vi "Find Unexpected Deps.vi"() -> ()   [LabVIEW 2019, in "DepsWatchToolsMenu.lvlib"]
doc: "GUI to compare LabVIEW code between currently checked out branch with any other branch or any of its commits.\n\n(c) 2024 Soliton Technologies. All rights reserved."
uses:
  DepsWatchToolsMenu.lvlib
  <vilib>/Hampel Software Engineering/Git API/Git API/GIT-api.lvclass
  <vilib>/Hampel Software Engineering/Git API/Git API/Controls/GIT-Repository States.ctl
  vi.lib/DepsWatch/DepsWatch.lvlib
  <userlib>/_OpenG.lib/file/file.llb/Valid Path - Traditional__ogtk.vi
  <userlib>/_OpenG.lib/file/file.llb/File Exists - Scalar__ogtk.vi
  vi.lib/DepsWatch/Typedefs/DepsCheckResult.ctl
panel:
  in  "Tab Control":T1(tab)=enum."Main UI"
  in  "Check Changed Libraries Only?":bool
  in  "Branch 2":string(combo)="origin/main" caption="Branch2 to Compare"
  in  "Refresh Current Branch":bool
  in  "Stop":bool
  in  "Repository Path":path
  in  "Branch1":string(combo)="origin/main" caption="Branch1 to Compare"
  in  "Compare":bool
  out "Current Branch Status":string
  out "Unexpected Deps":T2[](array[typedef])
  # "1. Checkout the branch of interest in your system using any method - Git command line, Desktop Git GUI Clients etc.,\n\n2. Specify the local Repository Path.\n\n3. Verify the current branch, its status and select a branch or commit based on the Compare Mode and click on Compare to display the file changes.\n\n4. Double click on a file to initiate LabVIEW code comparison.\n\n5. Once done with required comparisons, exit the tool by closing the window. The tool cleans up the temporary files added during comparison.\n\n\nNote:\n1. This tool uses LabVIEW's VI Comparison Tool which requires LabVIEW Professional Development System.\n2. It is recommended to not use other Git Clients actively when comparing files using this tool to avoid Git command related errors.\n3. It is recommended to commit all changes (working copy) before using this tool for comparison."
  # "This tool uses git diff command to identify the changes. Hence it is recommended to commit all the changes (working copy) to have them considered for comparison. For code comparison, this tool uses LabVIEW's built in VI Comparison Tool.\n\nExample: Identify changes in current branch when comparing with other branch\n\n---A---B---C---D    <== other branch\n               \\\n                 E---F      <== current branch\n\n1. We will need to identify only the file changes introduced by current branch. E and F commits are those changes in the above example (commits after the common ancestor B).\n2. For the identified file changes compare with the other branch (D) to see how it differs. These differences will be our current branch changelist.\n\nWhy only current branch changes?\nIt is most useful to see how the current branch will modify the files when it is getting merged. Best use case for displaying only current branch changelist will be for Pull Request reviews."
  # "1. Repository Path - Local repository path (the top level folder with '.git' hidden folder in it). Git API will be initialized for this repository.\n\n2. Current Branch - Currently checked out branch. The status of the current branch is also displayed at top right. Click Refresh button to update the current branch if it is changed in the system or received new changes via Git Pull.\n\n3. Compare Mode - Select the type of comparison. You can compare the current branch with another branch or with a particular commit of a selected branch.\n\nIn branch comparison mode, you can enter the branch name for comparison in Branch to Compare. Remote branches usually start with \"origin/\" and local branches do not have \"origin/\" prefix. The branch's recent commit is displayed in Recent Commit and its details in Commit Details for reference. \n\nIn commit comparison mode, the commits available in the branch selected in Select Branch are listed in Commit to Compare. For the commit selected in Commit to Compare, its details will be displayed in the Commit Details. Use Commits to Fetch to limit the number of commits obtained and improve the loading time.\n\n     Note: Git doesn't maintain information on when the branch is created. So, all the commits of the selected branch will be displayed (all the way up to the very first commit after repository creation). Without a limit, it increases loading time.\n\n4. Compare - Identifies the file changes and Current Branch Changelist table shows the list of all files that are different in the current branch compared to the branch/commit selected.\n\n     Note: The other branch/commit in comparison would have introduced its own changes that are not part of current branch. Those changes will not be displayed.\n\n5. Filter LabVIEW VI and Control Files - Filter files except VI and CTL files. These require LabVIEW to compare but project, library and classes are text files that can be easily reviewed in the desktop Git GUI clients or in Pull Request of Git web services.\n\n6. LabVIEW Compare Options - Options to decide what to compare in the code. Set the required options before initiating code compare.\n\n7. Double click on the file you wish to compare. LabVIEW opens the compare window for the file from the current branch and the file from the other branch/commit (file will be suffixed with TEMP). It may take a while if the VI/CTL have lot of dependencies to load. Having the project pre-opened and opening this tool from that instance may reduce the loading time. Note that the file from the other branch/commit in comparison may be missing its dependent files which may not be available in the current branch or deleted in the current branch commits. This will cause the file to be in a broken state but does not affect the comparison. Another reason for the broken state may be due to the parent library/class not recognizing this new file with the suffix but this as well will not affect the comparison.\n\n     Note: The files from other branch/commit are placed at the same location in the current branch so that the LabVIEW can load the dependencies appropriately.\n\n8. Viewed Status (mixed checkbox) - A tick mark appears for every file compared or opened. Use the mixed checkbox (below the Current Branch Changelist) to control status for all files.\n\n     Note: Viewed status is only a visual aid for tracking and does not have any other function other than that.\n\n9. Panel Close - Stops the tools execution after removing all the new files introduced into the current branch (TEMP files)."
  # "This GUI helps identify unexpected dependencies across all libraries in a repository. It also supports branch-to-branch comparison, allowing users to analyze dependency changes between any two branches and validate dependencies only for the modified libraries."
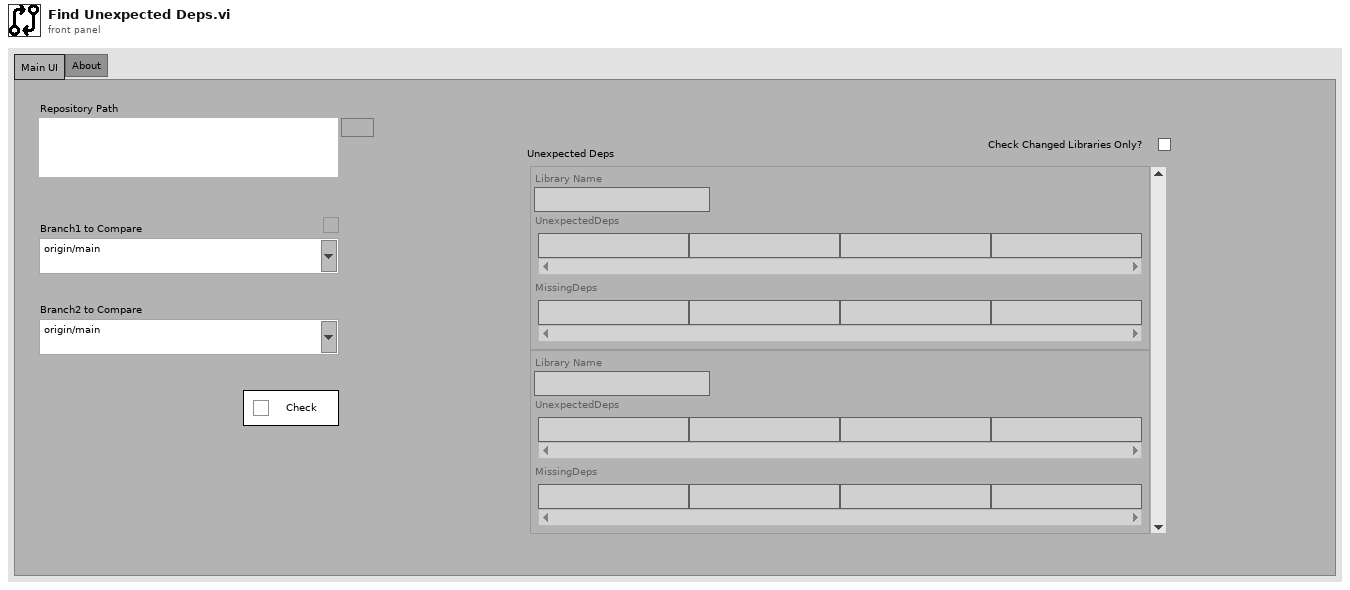
[diagram p1: front panel]
types:
  T1 = enum32{"Getting Started", "How it Works?", "Main UI", "Help", "About"}
  T2 = typedef "DepsWatch.lvlib/DepsCheckResult.ctl" = cluster{"Library Name":string, "UnexpectedDeps":string[], "MissingDeps":string[]}
  T3 = cluster{"Repository Path":path, "Git API Object":refnum<class "GIT-api.lvclass">, "Git API Initialized?":bool, "Current Branch":string, "Branch1 to Compare":string, "Branch2 to Compare":string, "Check Changed Libraries Only?":bool, "Failures":T2[]}
  T4 = enum8{"Enabled", "Disabled", "Disabled and Grayed Out"}
  T5 = typedef "GIT-API-for-LabVIEW.lvlib/GIT-api.lvclass/GIT-Repository States.ctl" = enum16{"up-to-date", "behind", "ahead", "diverged", "unpublished", "detached", "unknown"}
  T6 = typedef "DepsWatch.lvlib/CICDPathConfigs.ctl" = cluster{"GlobalIncludePaths":path[], "GlobalExcludePaths":path[], "BuildSpecsIncludePaths":path[], "ActualDepsIncludePaths":path[], "WorkspacePath":path, "SourceFolderPaths":path[], "ChangedFilesLogpaths":map{string, path}}
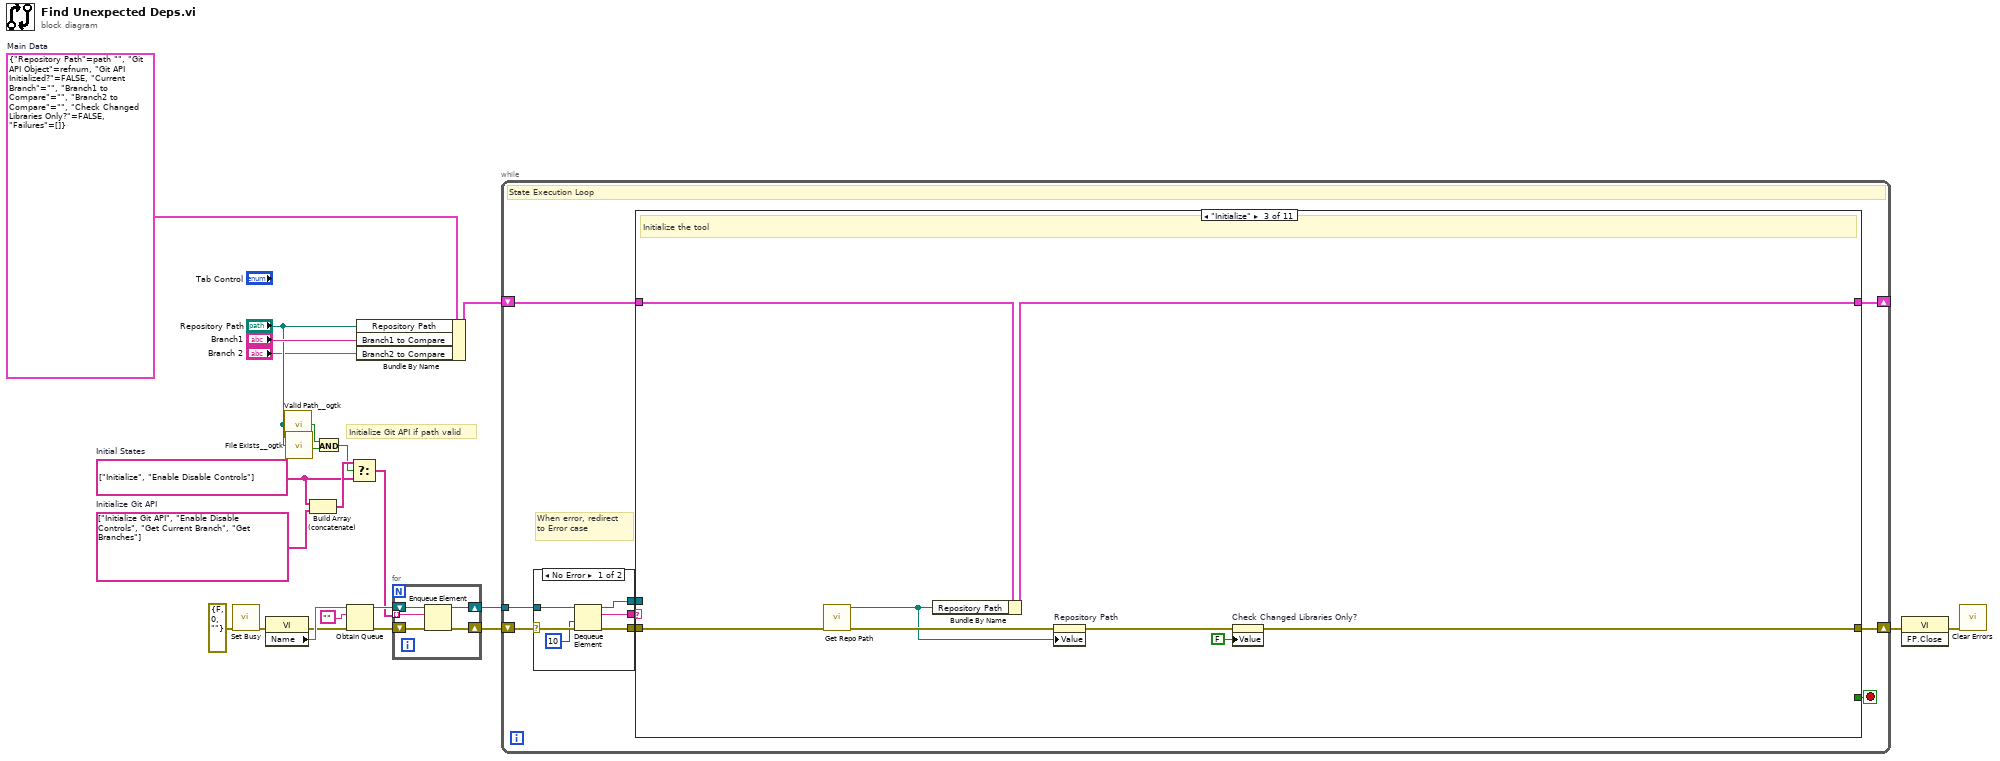
[diagram p0: block diagram]
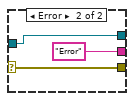
[diagram p2: hidden frame]
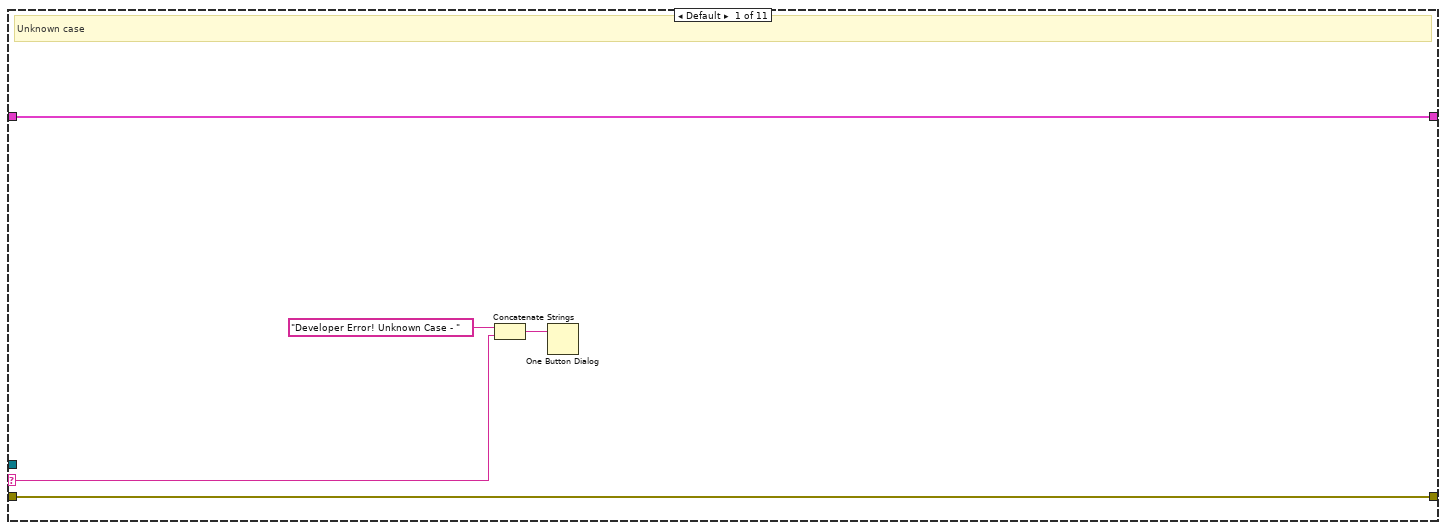
[diagram p3: hidden frame]
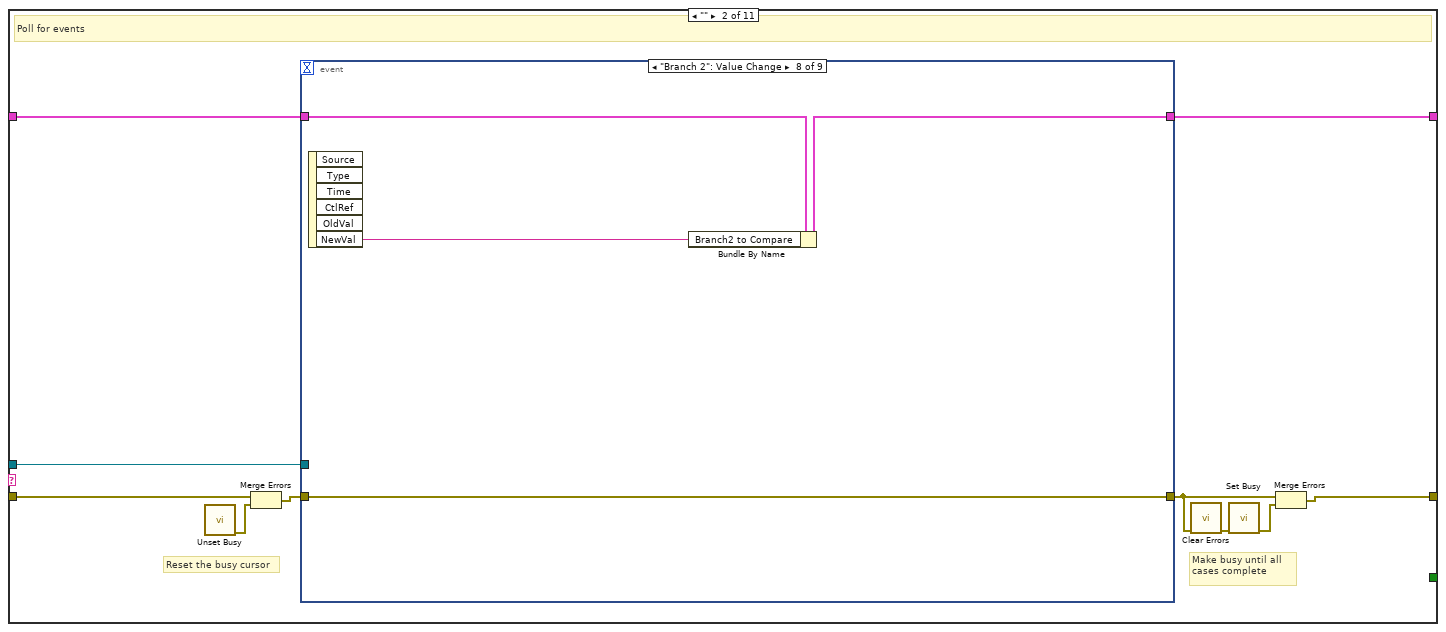
[diagram p4: hidden frame]
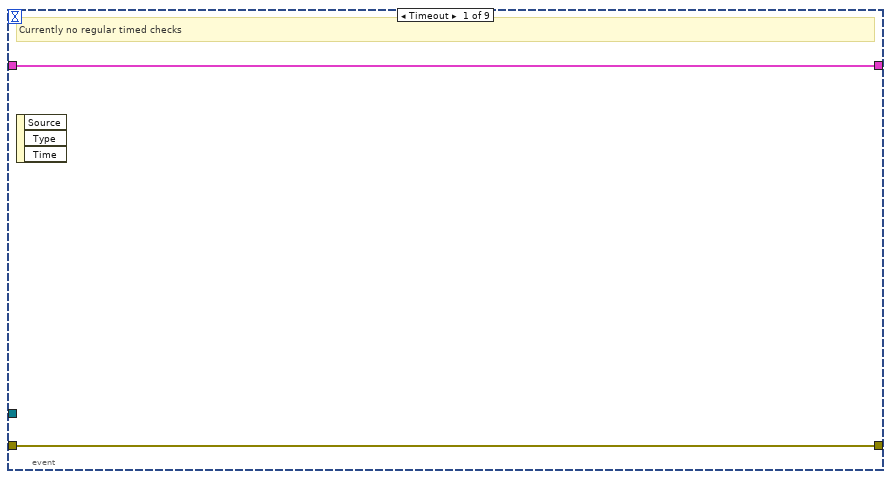
[diagram p5: hidden frame]
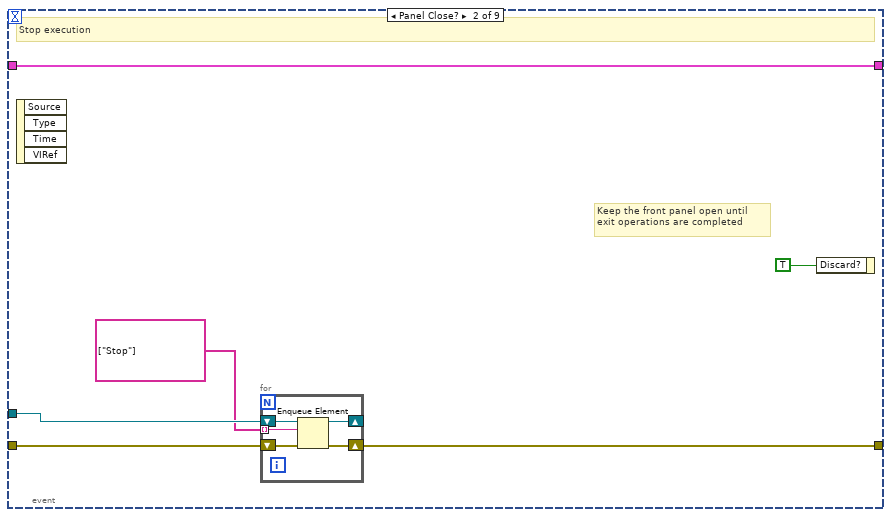
[diagram p6: hidden frame]
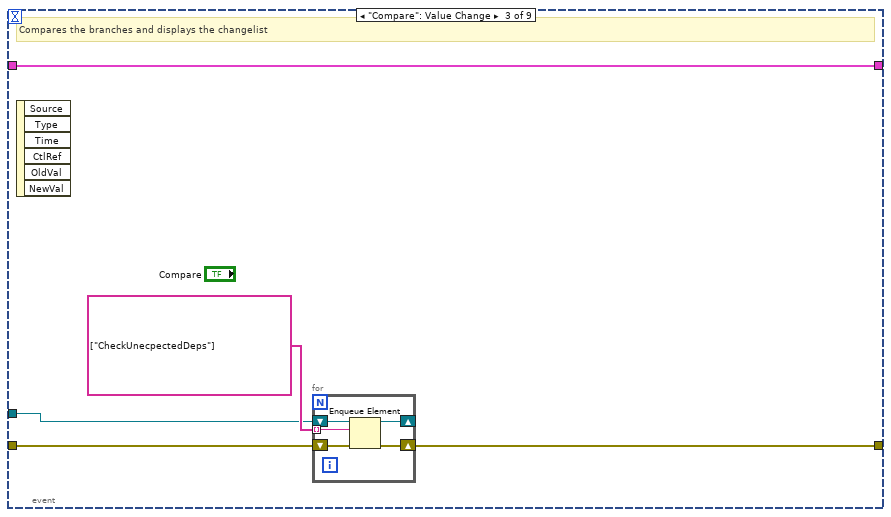
[diagram p7: hidden frame]
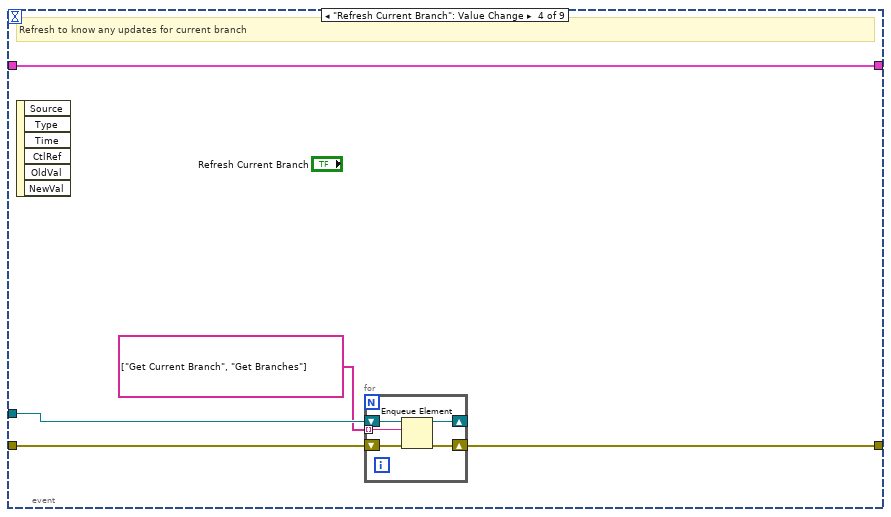
[diagram p8: hidden frame]
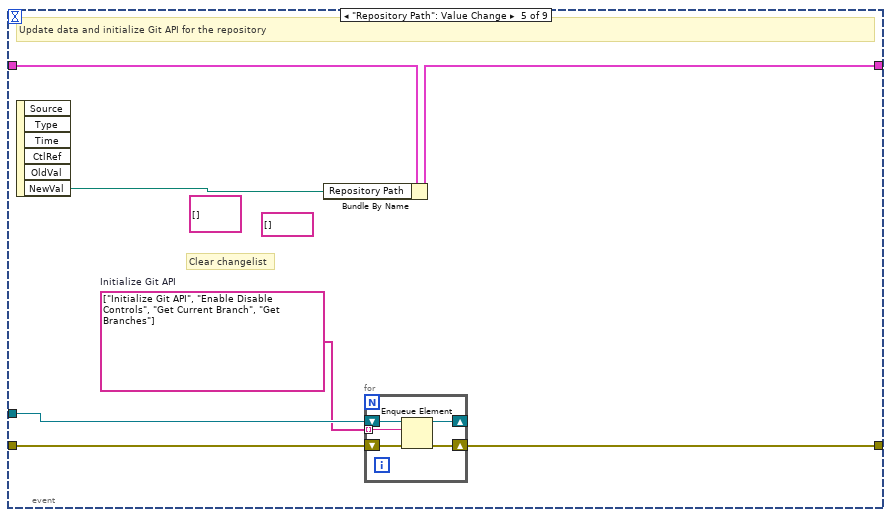
[diagram p9: hidden frame]
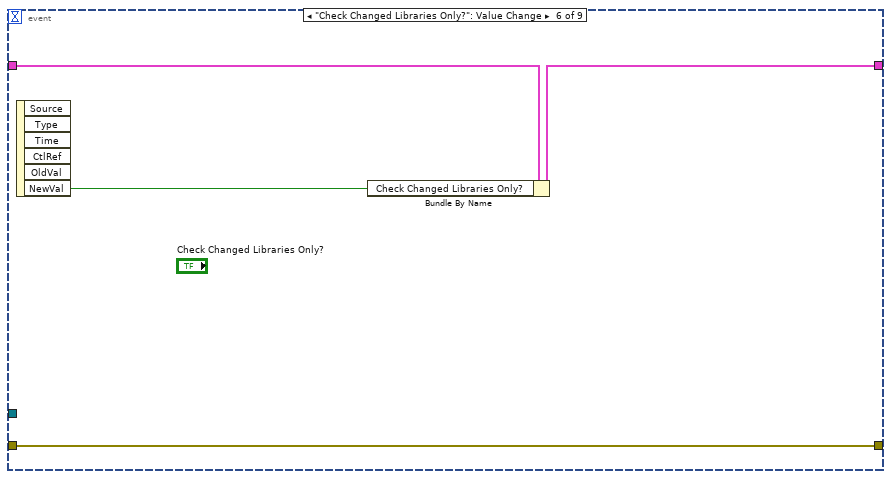
[diagram p10: hidden frame]
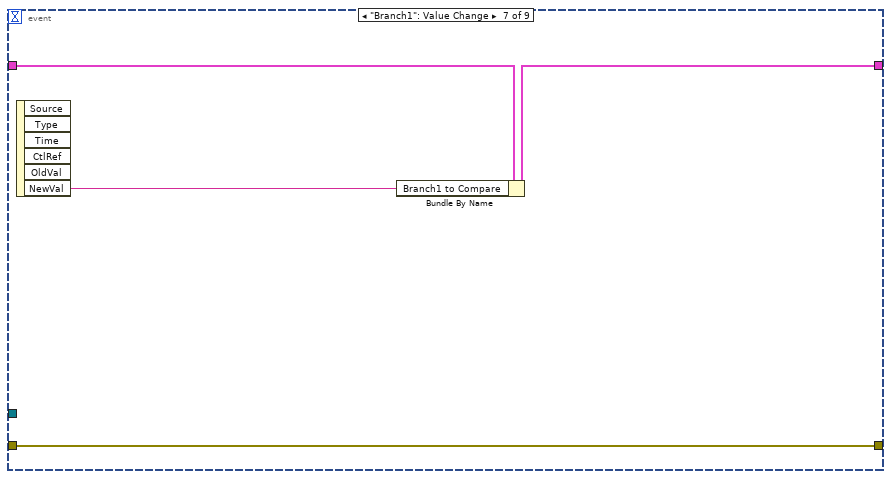
[diagram p11: hidden frame]
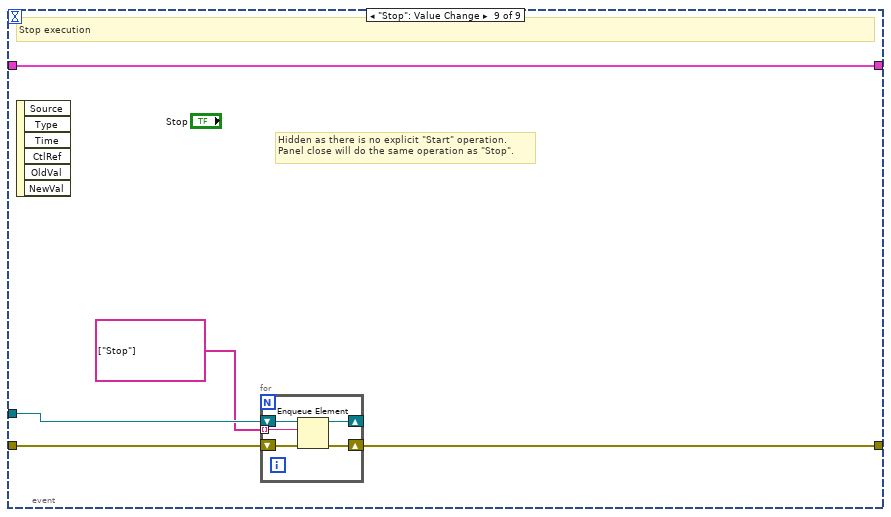
[diagram p12: hidden frame]
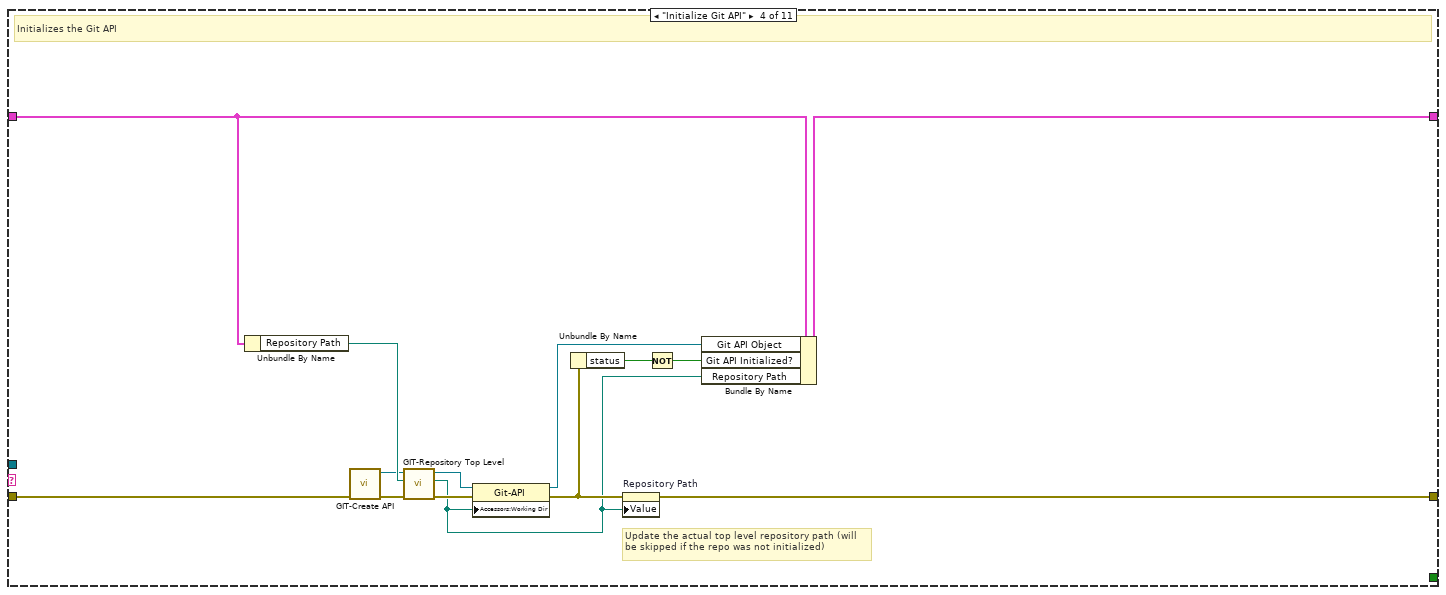
[diagram p13: hidden frame]
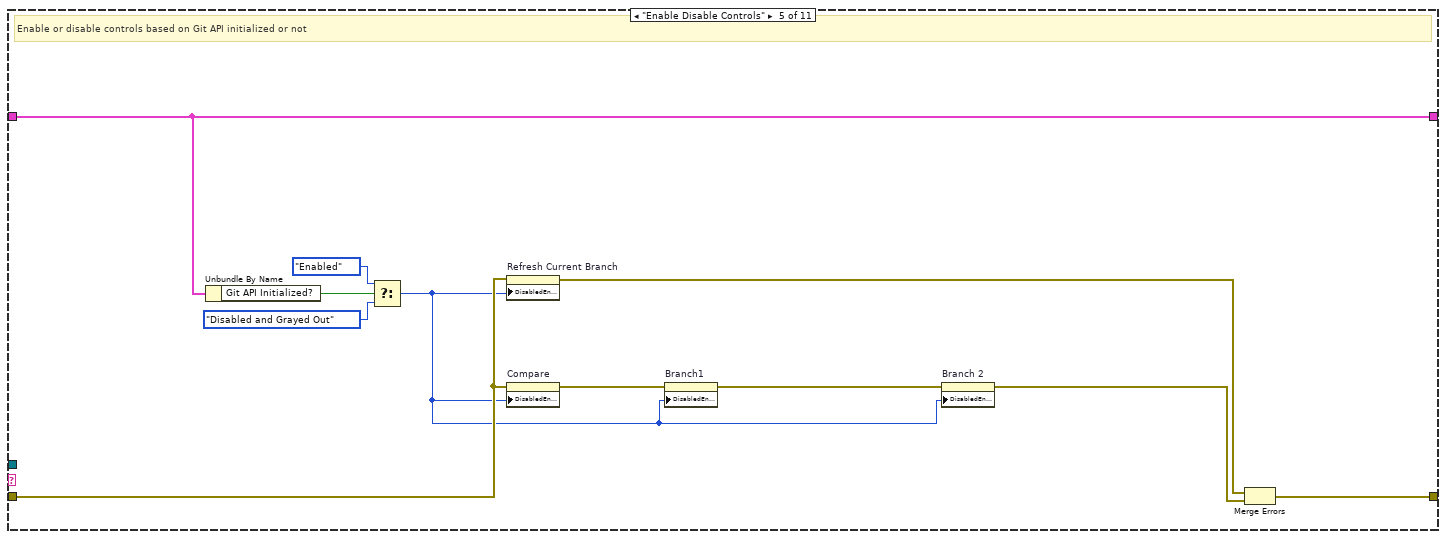
[diagram p14: hidden frame]
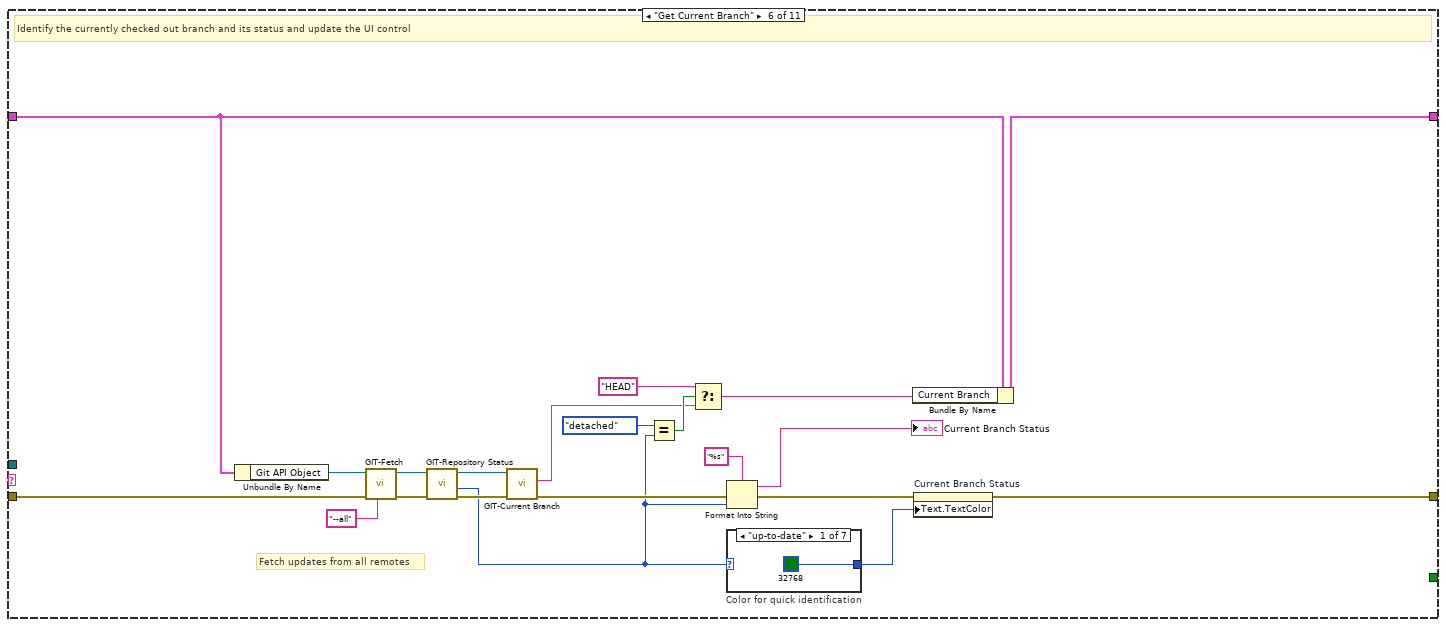
[diagram p15: hidden frame]
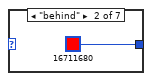
[diagram p16: hidden frame]
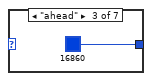
[diagram p17: hidden frame]
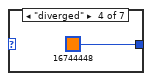
[diagram p18: hidden frame]
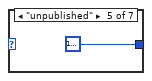
[diagram p19: hidden frame]
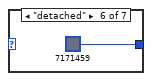
[diagram p20: hidden frame]
diagram:
  w13 = string[] ["Initialize Git API", "Enable Disable Controls", "Get Current Branch", "Get Branches"]  # Initialize Git API
  w11 = string[] ["Initialize", "Enable Disable Controls"]  # Initial States
  w20 = T3 {"Repository Path"=path "", "Git API Object"=refnum, "Git API Initialized?"=FALSE, "Current Branch"="", "Branch1 to Compare"="", "Branch2 to Compare"="", "Check Changed Libraries Only?"=FALSE, "Failures"=[]}  # Main Data
  # "Initialize Git API if path valid"
  n1 = call <vilib>:"Set Busy.vi"("error in (no error)"=errorcluster {"status"=FALSE, "code"=0, "source"=""}) -> ("error out"=w5:errorcluster)  [unwired: 9 in, 1 out]
  n2 = property class="VI"(error in=w5) -> (error out=w22:errorcluster, "Name"=w23:string)  [unwired: 1 in, 1 out]
  n3 = call-poly <userlib>:"Valid Path__ogtk.vi"("path"="Repository Path") -> ("valid"=w8:bool)
  n4 = call-poly <userlib>:"File Exists__ogtk.vi"("file path"="Repository Path") -> ("exists"=w9:bool)  [unwired: 6 in, 1 out]
  n5 = Build Array (concatenate)(w11, w13) -> (w12:string[])
  n6 = And(x=w8, y=w9) -> (x .and. y?=w7:bool)
  n7 = Obtain Queue(name (unnamed)=w23, element data type="", error in (no error)=w22) -> (queue out=w17:refnum<queue>, error out=w14:errorcluster)  [unwired: 2 in, 1 out]
  n8 = Select(t=w12, s=w7, f=w11) -> (s? t:f=w10:string[])
  n9 = Bundle By Name(cluster=w20, "Repository Path"="Repository Path", "Branch1 to Compare"="Branch1", "Branch2 to Compare"="Branch 2") -> (w19:T3)
  n10 = for {
    tunnel: w10 -> [w25] mode=indexing
    shift-right: [w27] -> w16
    shift-left: w14 -> [w28]
    shift-right: [w24] -> w15
    shift-left: w17 -> [w26]
    n11 = Enqueue Element(queue=w26, element=w25, error in (no error)=w28) -> (queue out=w24:refnum<queue>, error out=w27:errorcluster)  [unwired: 1 in, 1 out]
  }
  n12 = while {
    shift-right: [w29] -> w3
    shift-left: w16 -> [w31]
    tunnel: w15 -> [w32]
    shift-right: [w34] -> _
    shift-left: w19 -> [w33]
    stop <- w35 stop-if-true
    # "When error, redirect to Error case"
    # "State Execution Loop"
    n13 = case shown="No Error" w31 {
      selector: w31 -> [w40 w44]
      tunnel: [w43 "Error" ("element")] -> w37
      tunnel: [w42 w46] -> w36
      tunnel: w32 -> [w41 w46]
      tunnel: [w38 w44] -> w30
      frame No Error {
        n14 = Dequeue Element(queue=w41, timeout in ms (-1)=10, error in (no error)=w40) -> (queue out=w42:refnum<queue>, element=w43:string, error out=w38:errorcluster)  [unwired: 1 out]
      }
      frame Error {
      }
    }
    n15 = case shown="\"Initialize\"" w37 {
      selector: w37 -> [w50 _ _ _ _ _ _ _ _ _ _]
      tunnel: w30 -> [w48 w55 w132 w150 w154 w167 w194 w235 w260 w272 w280]
      tunnel: w36 -> [_ w61 _ _ _ _ _ _ w258 w269 w277]
      tunnel: [w48 w57 w135 w138 w156 w176 w195 w244 w259 w267 w273] -> w29
      tunnel: [_ _ _ _ _ _ _ _ _ w270 _] -> w35
      tunnel: [w47 w59 w131 w147 w161 w179 w193 w242 w257 w271 w281] -> w34
      tunnel: w33 -> [w47 w60 w136 w149 w161 w180 w198 w243 w257 w271 w281]
      frame Default {
        # "Unknown case"
        n16 = Concatenate Strings("Developer Error! Unknown Case - " ("string"), w50) -> (w49:string)
        n17 = One Button Dialog(message=w49) -> ()  [unwired: 1 in, 1 out]
      }
      frame "" {
        # "Reset the busy cursor"
        # "Make busy until all cases complete"
        # "Poll for events"
        n18 = call <vilib>:"Unset Busy.vi"() -> ("error out"=w56:errorcluster)  [unwired: 11 in]
        n19 = Merge Errors(w55, w56) -> (w54:errorcluster)
        n20 = event shown="[7] \"Branch 2\": Value Change" {
          selector: _ -> [_ _ _ _ _ _ _ _ _]
          dyn-events: _ -> [_ _ _ _ _ _ _ _ _]
          timeout: _ -> [_ _ _ _ _ _ _ _ _]
          tunnel: w54 -> [w62 w69 w78 w89 w98 w110 w114 w118 w123]
          tunnel: w61 -> [_ w68 w77 w88 w97 _ _ _ w122]
          tunnel: [w62 w67 w76 w86 w96 w110 w114 w118 w121] -> w53
          tunnel: w60 -> [w63 w66 w75 w85 w101 w109 w113 w117 w120]
          tunnel: [w63 w66 w75 w85 w100 w108 w112 w116 w120] -> w59
          event Timeout {
            # "Currently no regular timed checks"
            n21 = event-data() -> ()  [unwired: 1 in, 3 out]
          }
          event Panel Close? {
            # "Keep the front panel open until exit operations are completed"
            # "Stop execution"
            n22 = event-data() -> ()  [unwired: 1 in, 4 out]
            n23 = for {
              tunnel: string[] ["Stop"] -> [w71] mode=indexing
              shift-right: [w73] -> w67
              shift-left: w69 -> [w74]
              shift-right: [w70] -> _
              shift-left: w68 -> [w72]
              n24 = Enqueue Element(queue=w72, element=w71, error in (no error)=w74) -> (queue out=w70:refnum<queue>, error out=w73:errorcluster)  [unwired: 1 in, 1 out]
            }
            n25 = event-data("Discard?"=TRUE) -> ()  [unwired: 1 in, 1 out]
          }
          event "Compare": Value Change {
            # "Compares the branches and displays the changelist"
            n26 = event-data() -> ()  [unwired: 1 in, 6 out]
            n27 = for {
              tunnel: string[] ["CheckUnecpectedDeps"] -> [w81] mode=indexing
              shift-right: [w83] -> w76
              shift-left: w78 -> [w84]
              shift-right: [w80] -> _
              shift-left: w77 -> [w82]
              n28 = Enqueue Element(queue=w82, element=w81, error in (no error)=w84) -> (queue out=w80:refnum<queue>, error out=w83:errorcluster)  [unwired: 1 in, 1 out]
            }
          }
          event "Refresh Current Branch": Value Change {
            # "Refresh to know any updates for current branch"
            n29 = event-data() -> ()  [unwired: 1 in, 6 out]
            n30 = for {
              tunnel: string[] ["Get Current Branch", "Get Branches"] -> [w91] mode=indexing
              shift-right: [w93] -> w86
              shift-left: w89 -> [w94]
              shift-right: [w90] -> _
              shift-left: w88 -> [w92]
              n31 = Enqueue Element(queue=w92, element=w91, error in (no error)=w94) -> (queue out=w90:refnum<queue>, error out=w93:errorcluster)  [unwired: 1 in, 1 out]
            }
          }
          event "Repository Path": Value Change {
            w95 = string[] ["Initialize Git API", "Enable Disable Controls", "Get Current Branch", "Get Branches"]  # Initialize Git API
            (unwired) string[] [] ("Viewed Files")
            (unwired) string[][] [] ("Item Names")
            # "Clear changelist"
            # "Update data and initialize Git API for the repository"
            n32 = event-data() -> ("NewVal"=w99:path)  [unwired: 1 in, 5 out]
            n33 = Bundle By Name(cluster=w101, "Repository Path"=w99) -> (w100:T3)
            n34 = for {
              tunnel: w95 -> [w103] mode=indexing
              shift-right: [w105] -> w96
              shift-left: w98 -> [w106]
              shift-right: [w102] -> _
              shift-left: w97 -> [w104]
              n35 = Enqueue Element(queue=w104, element=w103, error in (no error)=w106) -> (queue out=w102:refnum<queue>, error out=w105:errorcluster)  [unwired: 1 in, 1 out]
            }
          }
          event "Check Changed Libraries Only?": Value Change {
            n36 = event-data() -> ("NewVal"=w107:bool)  [unwired: 1 in, 5 out]
            n37 = Bundle By Name(cluster=w109, "Check Changed Libraries Only?"=w107) -> (w108:T3)
          }
          event "Branch1": Value Change {
            n38 = event-data() -> ("NewVal"=w111:string)  [unwired: 1 in, 5 out]
            n39 = Bundle By Name(cluster=w113, "Branch1 to Compare"=w111) -> (w112:T3)
          }
          event "Branch 2": Value Change {
            n40 = event-data() -> ("NewVal"=w115:string)  [unwired: 1 in, 5 out]
            n41 = Bundle By Name(cluster=w117, "Branch2 to Compare"=w115) -> (w116:T3)
          }
          event "Stop": Value Change {
            # "Hidden as there is no explicit \"Start\" operation.\nPanel close will do the same operation as \"Stop\"."
            # "Stop execution"
            n42 = event-data() -> ()  [unwired: 1 in, 6 out]
            n43 = for {
              tunnel: string[] ["Stop"] -> [w125] mode=indexing
              shift-right: [w127] -> w121
              shift-left: w123 -> [w128]
              shift-right: [w124] -> _
              shift-left: w122 -> [w126]
              n44 = Enqueue Element(queue=w126, element=w125, error in (no error)=w128) -> (queue out=w124:refnum<queue>, error out=w127:errorcluster)  [unwired: 1 in, 1 out]
            }
          }
        }
        n45 = call <vilib>:"Clear Errors.vi"("error in (no error)"=w53) -> ("error out"=w52:errorcluster)  [unwired: 5 in, 1 out]
        n46 = call <vilib>:"Set Busy.vi"("error in (no error)"=w52) -> ("error out"=w58:errorcluster)  [unwired: 9 in, 1 out]
        n47 = Merge Errors(w53, w58) -> (w57:errorcluster)
      }
      frame "Initialize" {
        # "Initialize the tool"
        n48 = call "Get Repo Path.vi"("error in (no error)"=w132) -> ("error out"=w133:errorcluster, "Repo Path"=w129:path)  [unwired: 9 in]
        n49 = Bundle By Name(cluster=w136, "Repository Path"=w129) -> (w131:T3)
        n50 = property on="Repository Path" class="Path"(error in=w133, "Value"=w129) -> (error out=w130:errorcluster)  [unwired: 1 in, 1 out]
        n51 = property on="Check Changed Libraries Only?" class="Bool (strict)"(error in=w130, "Value"=FALSE ("Check Changed Libraries Only?")) -> (error out=w135:errorcluster)  [unwired: 1 in, 1 out]
      }
      frame "Initialize Git API" {
        # "Update the actual top level repository path (will be skipped if the repo was not initialized)"
        # "Initializes the Git API"
        n52 = Unbundle By Name(w149) -> ("Repository Path"=w146:path)
        n53 = call <vilib>:"GIT-Create API.vi"("error in"=w150) -> ("error out"=w145:errorcluster, "git-api out"=w143:refnum<class "GIT-api.lvclass">)  [unwired: 9 in]
        n54 = call <vilib>:"GIT-Repository Top Level.vi"("error in"=w145, "Current Path"=w146, "git-api in"=w143) -> ("error out"=w142:errorcluster, "Repo Top Level Path"=w137:path, "git-api out"=w144:refnum<class "GIT-api.lvclass">)  [unwired: 6 in]
        n55 = property class="Git-API"(reference=w144, error in=w142, "Accessors:Working Dir"=w137) -> (reference out=w148:refnum<class "GIT-api.lvclass">, error out=w139:errorcluster)
        n56 = Unbundle By Name(w139) -> ("status"=w141:bool)
        n57 = property on="Repository Path" class="Path"(error in=w139, "Value"=w137) -> (error out=w138:errorcluster)  [unwired: 1 in, 1 out]
        n58 = Not(x=w141) -> (.not. x?=w140:bool)
        n59 = Bundle By Name(cluster=w149, "Git API Object"=w148, "Git API Initialized?"=w140, "Repository Path"=w137) -> (w147:T3)
      }
      frame "Enable Disable Controls" {
        # "Enable or disable controls based on Git API initialized or not"
        n60 = Unbundle By Name(w161) -> ("Git API Initialized?"=w160:bool)
        n61 = Select(t=T4."Enabled" ("Disabled"), s=w160, f=T4."Disabled and Grayed Out" ("Disabled")) -> (s? t:f=w151:T4)
        n62 = property on="Refresh Current Branch" class="Bool"(error in=w154, "DisabledEnum"=w151) -> (error out=w157:errorcluster)  [unwired: 1 in, 1 out]
        n63 = property on="Compare" class="Bool"(error in=w154, "DisabledEnum"=w151) -> (error out=w155:errorcluster)  [unwired: 1 in, 1 out]
        n64 = property on="Branch1" class="CmbBox"(error in=w155, "DisabledEnum"=w151) -> (error out=w153:errorcluster)  [unwired: 1 in, 1 out]
        n65 = property on="Branch 2" class="CmbBox"(error in=w153, "DisabledEnum"=w151) -> (error out=w152:errorcluster)  [unwired: 1 in, 1 out]
        n66 = Merge Errors(w157, w152) -> (w156:errorcluster)
      }
      frame "Get Current Branch" {
        # "Fetch updates from all remotes"
        # "Identify the currently checked out branch and its status and update the UI control"
        n67 = Unbundle By Name(w180) -> ("Git API Object"=w168:refnum<class "GIT-api.lvclass">)
        n68 = call <vilib>:"GIT-Fetch.vi"("param"="--all", "error in"=w167, "git-api in"=w168) -> ("error out"=w173:errorcluster, "git-api out"=w174:refnum<class "GIT-api.lvclass">)  [unwired: 6 in, 1 out]
        n69 = call <vilib>:"GIT-Repository Status.vi"("error in"=w173, "git-api in"=w174) -> ("error out"=w182:errorcluster, "State"=w165:T5, "git-api out"=w181:refnum<class "GIT-api.lvclass">)  [unwired: 6 in, 1 out]
        n70 = call <vilib>:"GIT-Current Branch.vi"("error in"=w182, "git-api in"=w181) -> ("error out"=w166:errorcluster, "current branch"=w169:string)  [unwired: 6 in, 2 out]
        n71 = Equal?(x=GIT-Repository_States."detached", y=w165) -> (x = y?=w170:bool)
        n72 = Select(t="HEAD", s=w170, f=w169) -> (s? t:f=w164:string)
        n73 = Format Into String(format string="%s", error in=w166, w165) -> (resulting string=→"Current Branch Status":string, error out=w162:errorcluster)  [unwired: 1 in]
        n74 = case "Color for quick identification" shown="\"up-to-date\"" w165 {
          tunnel: [u32 32768 u32 16711680 u32 16860 u32 16744448 u32 16777222 u32 7171459 u32 16711680] -> w175
          frame "up-to-date" {
          }
          frame "behind" {
          }
          frame "ahead" {
          }
          frame "diverged" {
          }
          frame "unpublished" {
          }
          frame "detached" {
          }
          frame "unknown" {
          }
        }
        n75 = Bundle By Name(cluster=w180, "Current Branch"=w164) -> (w179:T3)
        n76 = property on="Current Branch Status" class="Str"(error in=w162, "Text.TextColor"=w175) -> (error out=w176:errorcluster)  [unwired: 1 in, 1 out]
      }
      frame "CheckUnecpectedDeps" {
        w200 = TRUE  # GUI Mode? {F)
        n77 = Unbundle By Name(w198) -> ("Repository Path"=w197:path, "Check Changed Libraries Only?"=w196:bool, "Branch1 to Compare"=w191:string, "Branch2 to Compare"=w190:string)
        n78 = case shown="True" w196 {
          tunnel: [w201 w212] -> w199
          tunnel: w200 -> [_ w211]
          tunnel: w197 -> [_ w206]
          tunnel: w194 -> [w201 w205]
          tunnel: w191 -> [_ w203]
          tunnel: w190 -> [_ w202]
          frame False {
          }
          frame True {
            # "Update Changed Libraries List."
            n79 = call "ReadCICDPathConfig.vi"("error in (no error)"=w205, "Workspace Path"=w206) -> ("error out"=w204:errorcluster, "CICD Path Config Out"=w210:T6)  [unwired: 8 in]
            n80 = Unbundle By Name(w210) -> ("ChangedFilesLogpaths"=w208:map{string, path})
            n81 = Look In Map(map=w208, key="InScopeChangedLVFilesPath") -> (value=w207:path)  [unwired: 1 in, 1 out]
            n82 = call "GenerateChangedFilesList.vi"("GUI Mode? {F)"=w211, "Output File Path"=w207, "error in (no error)"=w204, "Branch 2"=w202, "Branch 1"=w203, "Workspace Path"=w206) -> ("error out"=w213:errorcluster)  [unwired: 5 in]
            n83 = call "GenerateChangedLibrariesList.vi"("GUI Mode? {F)"=w211, "error in (no error)"=w213, "Workspace Path"=w206) -> ("error out"=w212:errorcluster)  [unwired: 8 in]
          }
        }
        n84 = call "UnexpectedDepsCheck.vi"("GUI Mode? {F)"=w200, "error in (no error)"=w199, "CheckChangedLibrariesOnly"=w196, "Workspace Path"=w197) -> ("error out"=w195:errorcluster, "Failures"=w192:T2[])  [unwired: 5 in, 1 out]
        "Unexpected Deps" <- w192
        n85 = Bundle By Name(cluster=w198, "Failures"=w192) -> (w193:T3)
      }
      frame "Get Branches" {
        w225 = 0  # Branch Name List
        w230 = string[][] []
        w229 = "%s" ("format string")
        # "Reset if previous value not found"
        # "Combine local and remote branches"
        # "List Local branches"
        # "List Remote branches\nNote: All remote branches usually start with origin/ unless renamed"
        # "Reset if previous value not found"
        # "Get all local and remote branches and update UI control"
        n86 = Unbundle By Name(w243) -> ("Git API Object"=w233:refnum<class "GIT-api.lvclass">, "Current Branch"=w214:string)
        n87 = call <vilib>:"GIT-Branch.vi"("error in"=w235, "git-api in"=w233) -> ("error out"=w234:errorcluster, "std out"=w226:string, "git-api out"=w227:refnum<class "GIT-api.lvclass">)  [unwired: 7 in]
        n88 = call <vilib>:"GIT-Branch.vi"("param"="-r", "error in"=w234, "git-api in"=w227) -> ("error out"=w237:errorcluster, "std out"=w228:string)  [unwired: 6 in, 1 out]
        n89 = Spreadsheet String To Array(format string=w229, spreadsheet string=w226, array type (2D Dbl)=w230) -> (array=w246:string[][])  [unwired: 1 in]
        n90 = Spreadsheet String To Array(format string=w229, spreadsheet string=w228, array type (2D Dbl)=w230) -> (array=w231:string[][])  [unwired: 1 in]
        n91 = Index Array(array=w246, index (col)=w225) -> (element=w232:string[])  [unwired: 1 in]
        n92 = Index Array(array=w231, index (col)=w225) -> (element=w221:string[])  [unwired: 1 in]
        n93 = for "Remove current branch pointer" {
          tunnel: w232 -> [w255] mode=indexing
          tunnel: [w251] -> w224 mode=indexing
          tunnel: [w250] -> w247 mode=indexing
          n94 = Search and Replace String(input string=w255, search string="*", replace string="") -> (result string=w252:string, error out=w250:errorcluster)  [unwired: 5 in, 2 out]
          n95 = call <vilib>:"Trim Whitespace.vi"("string"=w252) -> ("trimmed string"=w251:string)  [unwired: 1 in]
        }
        n96 = for {
          tunnel: [w249] -> w222 mode=indexing
          tunnel: w221 -> [w248] mode=indexing
          n97 = call <vilib>:"Trim Whitespace.vi"("string"=w248) -> ("trimmed string"=w249:string)  [unwired: 1 in]
        }
        n98 = Build Array (concatenate)(w224, w222) -> (w215:string[])
        n99 = Search 1D Array(1D array=w215, element=w214) -> (index of element=w217:i32)  [unwired: 1 in]
        n100 = Merge Errors(w237, w247) -> (w223:errorcluster)
        n101 = Greater Or Equal To 0?(x=w217) -> (x >= 0?=w218:bool)
        n102 = Select(t=w214, s=w218, f="") -> (s? t:f=w216:string)
        n103 = property on="Branch1" class="CmbBox"(error in=w223, "Strings[]"=w215, "Value"=w216) -> (error out=w245:errorcluster)  [unwired: 1 in, 1 out]
        n104 = property on="Branch 2" class="CmbBox"("Strings[]"=w215) -> ("Value"=w220:string)  [unwired: 2 in, 2 out]
        n105 = Search 1D Array(1D array=w215, element=w220) -> (index of element=w241:i32)  [unwired: 1 in]
        n106 = Greater Or Equal To 0?(x=w241) -> (x >= 0?=w240:bool)
        n107 = Select(t=w220, s=w240, f="") -> (s? t:f=w238:string)
        n108 = property on="Branch 2" class="CmbBox"(error in=w245, "Value"=w238) -> (error out=w244:errorcluster)  [unwired: 1 in, 1 out]
        n109 = Bundle By Name(cluster=w243, "Branch2 to Compare"=w238) -> (w242:T3)
      }
      frame "Stop" {
        # "Performs actions when the VI is stopped."
        n110 = for {
          tunnel: string[] ["Exit"] -> [w262] mode=indexing
          shift-right: [w264] -> w259
          shift-left: w260 -> [w265]
          shift-right: [w261] -> _
          shift-left: w258 -> [w263]
          n111 = Enqueue Element(queue=w263, element=w262, error in (no error)=w265) -> (queue out=w261:refnum<queue>, error out=w264:errorcluster)  [unwired: 1 in, 1 out]
        }
      }
      frame "Exit" {
        w270 = TRUE  # Exit?
        # "Remove the beta tag as we don't want to accidentally save the VI with the tag which will then show up in the Tools -> SLL Toolkit menu."
        # "Finish the execution"
        n112 = Release Queue(queue=w269, error in (no error)=w272) -> (error out=w268:errorcluster)  [unwired: 1 in, 2 out]
        n113 = property class="VI"(error in=w268, "Front Panel.Title"="SLL LabVIEW Code Compare Tool for Git" ("Front Panel Window:Title")) -> (error out=w267:errorcluster)  [unwired: 1 in, 1 out]
      }
      frame "Error" {
        # "In case of any Git API initialization errors, we need to disable the controls."
        # "Show the error dialog and clear out the operations. Update controls status."
        n114 = call <vilib>:"Simple Error Handler.vi"("error in (no error)"=w280) -> ("error out"=w279:errorcluster)  [unwired: 4 in, 4 out]
        n115 = call <vilib>:"Clear Errors.vi"("error in (no error)"=w279) -> ("error out"=w278:errorcluster)  [unwired: 5 in, 1 out]
        n116 = Flush Queue(queue=w277, error in (no error)=w278) -> (queue out=w274:refnum<queue>, error out=w275:errorcluster)  [unwired: 1 out]
        n117 = for {
          tunnel: string[] ["Enable Disable Controls"] -> [w283] mode=indexing
          shift-right: [w285] -> w273
          shift-left: w275 -> [w286]
          shift-right: [w282] -> _
          shift-left: w274 -> [w284]
          n118 = Enqueue Element(queue=w284, element=w283, error in (no error)=w286) -> (queue out=w282:refnum<queue>, error out=w285:errorcluster)  [unwired: 1 in, 1 out]
        }
      }
    }
  }
  n119 = invoke class="VI" method="FP.Close"(error in=w3) -> (error out=w2:errorcluster)  [unwired: 2 in, 2 out]
  n120 = call <vilib>:"Clear Errors.vi"("error in (no error)"=w2) -> ()  [unwired: 5 in, 2 out]
